vi "Basic Test A.vi"() -> ()   [LabVIEW 2017]
uses:
  <vilib>/myRIO/Instrument Drivers/Onboard IO/PWM/typedefs/PWM Reference.ctl
  <vilib>/myRIO/Common/Instrument Driver Framework/Utilities/typedefs/myRIO Generic Hardware Reference.ctl
  <vilib>/myRIO/Common/Instrument Driver Framework/Utilities/typedefs/Hardware Version Enum.ctl
  <vilib>/myRIO/Common/Instrument Driver Framework/Utilities/typedefs/myRIO v1.0 Reference.ctl
  <vilib>/myRIO/Common/Instrument Driver Framework/Utilities/typedefs/Generic FPGA Reference.ctl
  <vilib>/myRIO/Common/Instrument Driver Framework/myRIO v1.0/PWM/typedefs/PWM Channels Enum.ctl
  <vilib>/myRIO/Instrument Drivers/Onboard IO/PWM/typedefs/PWM Configuration.ctl
  <vilib>/userdefined/High Color/nirio_resource_hc.ctl
  <vilib>/myRIO/Common/Instrument Driver Framework/myRIO v1.0/Encoder/typedefs/Encoder Signal Mode.ctl
  <vilib>/myRIO/Instrument Drivers/Onboard IO/Encoder/typedefs/Encoder Reference.ctl
  <vilib>/myRIO/Common/Instrument Driver Framework/myRIO v1.0/Encoder/typedefs/Encoder Channels Enum.ctl
  <vilib>/myRIO/Common/Instrument Driver Framework/myRIO v1.0/Encoder/typedefs/Encoder Configuration v1.0.ctl
  <vilib>/myRIO/Common/Instrument Driver Framework/Utilities/vis/Is FPGA Ref Available.vi
  <vilib>/myRIO/Common/Instrument Driver Framework/myRIO v1.0/PWM/vis/myRIO v1.1 Open PWM.vi
  <vilib>/myRIO/Instrument Drivers/Onboard IO/PWM/vis/Set Duty Cycle and Frequency.vi
  <vilib>/myRIO/Common/Instrument Driver Framework/myRIO v1.0/Encoder/vis/myRIO v1.1 Open Encoder.vi
  <vilib>/myRIO/Instrument Drivers/Onboard IO/Encoder/vis/Read.vi
  <vilib>/myRIO/Common/Instrument Driver Framework/Utilities/vis/Validate Channels.vi
  <vilib>/myRIO/Common/Instrument Driver Framework/myRIO v1.0/PWM/vis/myRIO v1.0 Reserve PWM.vi
  <vilib>/myRIO/Common/Instrument Driver Framework/myRIO v1.0/Encoder/vis/myRIO v1.0 Reserve Encoder.vi
  <vilib>/myRIO/Common/Instrument Driver Framework/myRIO v1.0/PWM/vis/myRIO v1.0 Build MUX Configuration PWM.vi
  <vilib>/myRIO/Common/Instrument Driver Framework/myRIO v1.0/Resource Manager/vis/myRIO v1.0 Reserve Channel List.vi
  <vilib>/myRIO/Common/Instrument Driver Framework/myRIO v1.0/Encoder/vis/myRIO v1.0 Build MUX Configuration Encoder.vi
  <vilib>/myRIO/Common/Instrument Driver Framework/myRIO v1.0/Resource Manager/vis/myRIO v1.0 Create Configuration List.vi
  <vilib>/myRIO/Common/Instrument Driver Framework/myRIO v1.0/Resource Manager/vis/myRIO v1.0 Reserve Channel.vi
  <vilib>/myRIO/Common/Instrument Driver Framework/myRIO v1.0/Resource Manager/vis/myRIO v1.0 Unreserve Channel.vi
  <vilib>/myRIO/Common/Instrument Driver Framework/myRIO v1.0/Resource Manager/vis/myRIO v1.0 Build Mutex Name.vi
  <vilib>/Utility/VariantDataType/GetNumericInfo.vi
  <vilib>/Utility/error.llb/Error Cluster From Error Code.vi
  <vilib>/myRIO/Common/Instrument Driver Framework/myRIO v1.0/myRIO v1.1 Open.vi
  <vilib>/myRIO/Common/Instrument Driver Framework/Utilities/vis/IO Manager.vi
  <vilib>/myRIO/Common/Instrument Driver Framework/Utilities/vis/Configuration Manager.vi
  <vilib>/myRIO/Common/Instrument Driver Framework/myRIO v1.0/Resource Manager/vis/myRIO v1.0 Configure IO.vi
  <vilib>/myRIO/Common/Instrument Driver Framework/myRIO v1.0/myRIO v1.0 Close.vi
  <vilib>/myRIO/Common/Instrument Driver Framework/myRIO v1.0/PWM/vis/myRIO v1.0 Write PWM.vi
  <vilib>/myRIO/Common/Instrument Driver Framework/myRIO v1.0/Encoder/vis/myRIO v1.0 Configure Encoder.vi
  <vilib>/myRIO/Common/Instrument Driver Framework/myRIO v1.0/Encoder/vis/myRIO v1.0 Read Encoder.vi
  <vilib>/myRIO/Express VI/Onboard IO/PWM/PWM Express VI.xnode
  <vilib>/myRIO/Instrument Drivers/Onboard IO/PWM/vis/myRIO PWM Open.xnode
  <vilib>/myRIO/Express VI/Onboard IO/Encoder/Encoder Express VI.xnode
  <vilib>/myRIO/Common/Instrument Driver Framework/myRIO v1.0/Encoder/typedefs/Encoder Count Direction Enum.ctl
  <vilib>/myRIO/Instrument Drivers/Onboard IO/Encoder/vis/myRIO Encoder Open.xnode
  <vilib>/myRIO/Instrument Drivers/Onboard IO/PWM/PWM.lvlib
  <vilib>/myRIO/Instrument Drivers/Onboard IO/Encoder/Encoder.lvlib
panel:
  out "Counter Value D":i32
  out "Counter Direction 4":enum16{"Counting Up", "Counting Down"}(ring)
  out "Overflow? 4":bool
  in  "Duty Cycle In C1":dbl(slide)=-0.013927576601671307 scale=-1.0..1.0
  out "Counter Value C":i32
  out "Counter Direction 3":enum16{"Counting Up", "Counting Down"}(ring)
  out "Overflow? 3":bool
  in  "Duty Cycle In B0":dbl(slide)=-0.013927576601671307 scale=-1.0..1.0
  out "Counter Value B":i32
  out "Counter Direction 2":enum16{"Counting Up", "Counting Down"}(ring)
  out "Overflow? 2":bool
  in  "Duty Cycle In A1":dbl(slide)=-0.013927576601671307 scale=-1.0..1.0
  in  "stop":bool
  in  "Duty Cycle In A0":dbl(slide)=-0.013927576601671307 scale=-1.0..1.0
  out "Overflow?":bool
  out "Counter Direction":enum16{"Counting Up", "Counting Down"}(ring)
  out "Counter Value A":i32
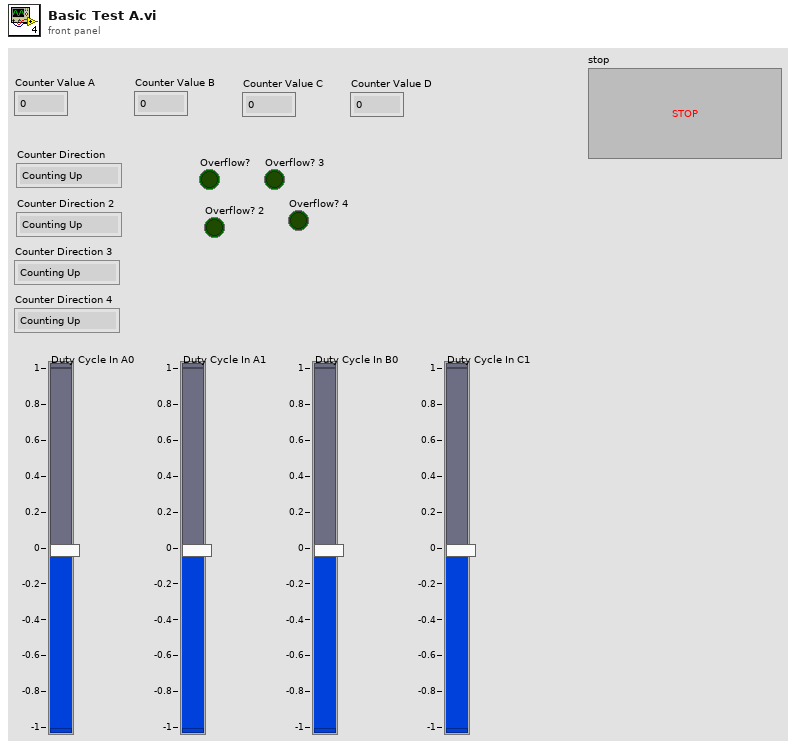
[diagram p1: front panel]
types:
  T1 = typedef "Encoder.lvlib/Encoder Reference.ctl" = cluster{"myRIO Reference":T2, "Encoder Channels Enum":T6}
  T2 = typedef "myRIO Generic Hardware Reference.ctl" = cluster{"myRIO Model":T3, "myRIO Hardware Reference":T4}
  T3 = typedef "Hardware Version Enum.ctl" = enum16{"Unknown", "myRIO-1900", "myRIO-1950", "roboRIO", "NI ELVIS RIO CM"}
  T4 = typedef "myRIO v1.0 Reference.ctl" = cluster{"Generic FPGA Reference":T5, "Allow multiple opens":bool}
  T5 = typedef "Generic FPGA Reference.ctl" = refnum<k20>
  T6 = typedef "Encoder Channels Enum.ctl" = enum16{"Not Connected", "C/ENC0", "C/ENC1", "A/ENC", "B/ENC", "DIO/ENC0", "DIO/ENC1", "DIO/ENC2", "DIO/ENC3", "DIO/ENC4"}
  T7 = typedef "Encoder Signal Mode.ctl" = enum16{"Quadrature phase signal", "Step and direction signal"}
  T8 = typedef "nirio_resource_hc.ctl" = tag
  T9 = typedef "PWM.lvlib/PWM Reference.ctl" = cluster{"myRIO Reference":T2, "PWM Channels Enum":T10, "PWM Configuration":T11}
  T10 = typedef "PWM Channels Enum.ctl" = enum16{"Not Connected", "C/PWM0", "C/PWM1", "A/PWM0", "A/PWM1", "A/PWM2", "B/PWM0", "B/PWM1", "B/PWM2", "PWM/PWM0", "PWM/PWM1", "PWM/PWM2", "PWM/PWM3", "PWM/PWM4", "PWM/PWM5", "PWM/PWM6", "PWM/PWM7", "PWM/PWM8", "PWM/PWM9"}
  T11 = typedef "PWM.lvlib/PWM Configuration.ctl" = cluster{"Frequency":dbl, "Duty Cycle":dbl}
  T12 = typedef "Encoder Count Direction Enum.ctl" = enum16{"Counting Up", "Counting Down"}
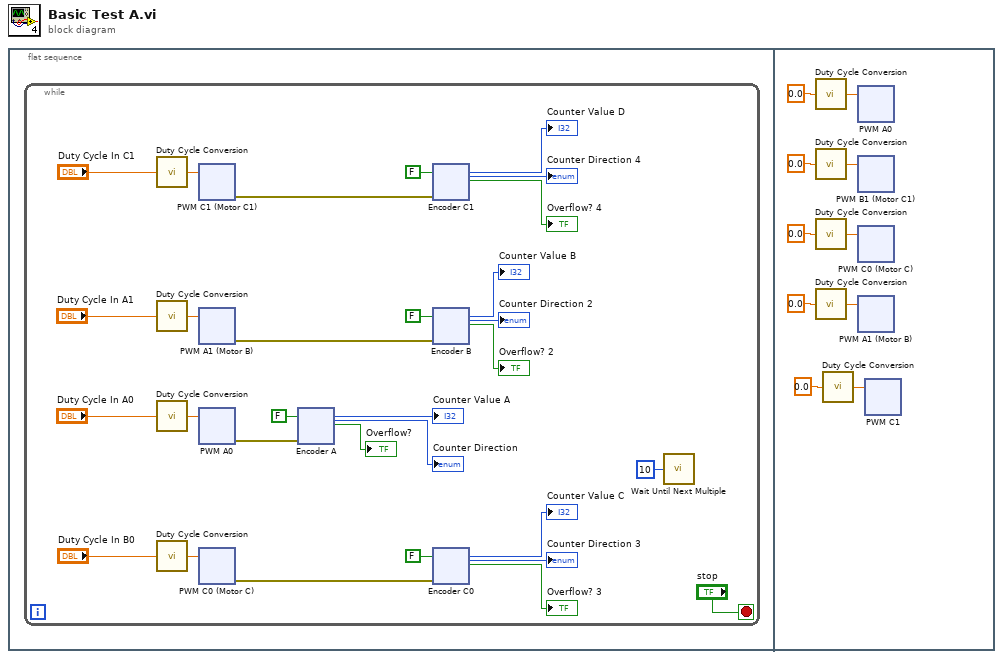
[diagram p0: block diagram]
diagram:
  n1 = flat-sequence {
    frame #0 {
      n2 = while {
        stop <- "stop" stop-if-true
        n3 = call "Duty Cycle Conversion.vi"("Duty Cycle In"="Duty Cycle In C1") -> ("Duty Cyle Out"=w2:dbl)
        n4 = call "Duty Cycle Conversion.vi"("Duty Cycle In"="Duty Cycle In A1") -> ("Duty Cyle Out"=w16:dbl)
        n5 = call "Duty Cycle Conversion.vi"("Duty Cycle In"="Duty Cycle In A0") -> ("Duty Cyle Out"=w30:dbl)
        n6 = call "Duty Cycle Conversion.vi"("Duty Cycle In"="Duty Cycle In B0") -> ("Duty Cyle Out"=w15:dbl)
        n7 = xnode "PWM C1 (Motor C1)"("Duty Cycle"=w2) -> ("error out"=w3:errorcluster)  [unwired: 1 in]
        n8 = xnode "PWM A1 (Motor B)"("Duty Cycle"=w16) -> ("error out"=w17:errorcluster)  [unwired: 1 in]
        n9 = xnode "PWM A0"("Duty Cycle"=w30) -> ("error out"=w29:errorcluster)  [unwired: 1 in]
        n10 = xnode "PWM C0 (Motor C)"("Duty Cycle"=w15) -> ("error out"=w14:errorcluster)  [unwired: 1 in]
        n11 = xnode "Encoder A"("error in (no error)"=w29, "Reset Counter"=FALSE) -> ("Counter Value"=→"Counter Value A":i32, "Counter Direction"=→"Counter Direction":T12, "Overflow?"=→"Overflow?":bool)  [unwired: 1 out]
        n12 = xnode "Encoder C1"("error in (no error)"=w3, "Reset Counter"=FALSE) -> ("Counter Value"=→"Counter Value D":i32, "Counter Direction"=→"Counter Direction 4":T12, "Overflow?"=→"Overflow? 4":bool)  [unwired: 1 out]
        n13 = xnode "Encoder B"("error in (no error)"=w17, "Reset Counter"=FALSE) -> ("Counter Value"=→"Counter Value B":i32, "Counter Direction"=→"Counter Direction 2":T12, "Overflow?"=→"Overflow? 2":bool)  [unwired: 1 out]
        n14 = xnode "Encoder C0"("error in (no error)"=w14, "Reset Counter"=FALSE) -> ("Counter Value"=→"Counter Value C":i32, "Counter Direction"=→"Counter Direction 3":T12, "Overflow?"=→"Overflow? 3":bool)  [unwired: 1 out]
        n15 = call "Wait Until Next Multiple"("Count(mSec)"=u32 10) -> ()  [unwired: 1 out]
      }
    }
    frame #1 {
      n16 = call "Duty Cycle Conversion.vi"("Duty Cycle In"=0.0) -> ("Duty Cyle Out"=w364:dbl)
      n17 = call "Duty Cycle Conversion.vi"("Duty Cycle In"=0.0) -> ("Duty Cyle Out"=w360:dbl)
      n18 = call "Duty Cycle Conversion.vi"("Duty Cycle In"=0.0) -> ("Duty Cyle Out"=w361:dbl)
      n19 = call "Duty Cycle Conversion.vi"("Duty Cycle In"=0.0) -> ("Duty Cyle Out"=w362:dbl)
      n20 = call "Duty Cycle Conversion.vi"("Duty Cycle In"=0.0) -> ("Duty Cyle Out"=w355:dbl)
      n21 = xnode "PWM A0"("Duty Cycle"=w364) -> ()  [unwired: 1 in, 1 out]
      n22 = xnode "PWM B1 (Motor C1)"("Duty Cycle"=w360) -> ()  [unwired: 1 in, 1 out]
      n23 = xnode "PWM C0 (Motor C)"("Duty Cycle"=w361) -> ()  [unwired: 1 in, 1 out]
      n24 = xnode "PWM A1 (Motor B)"("Duty Cycle"=w362) -> ()  [unwired: 1 in, 1 out]
      n25 = xnode "PWM C1"("Duty Cycle"=w355) -> ()  [unwired: 1 in, 1 out]
    }
  }
